vi "setKey.vi"(7 "LegendProperties":T1={"Appearance"={"layout"="", "text-sample order"="", "key order"="", "surroundingBox"=""}, "Alignment"={"Horizontal"="", "Vertical"=""}, "Location"="auto", "\"At\" location"={"XcoordSys"="", "YcoordSys"="", "Xvalue"=0.0, "Yvalue"=0.0}}, 8 "Set?":bool=TRUE, 11 "String in":string) -> (2 "command":string, 3 "String out":string)   [LabVIEW 2013]
uses:
  legendProperties.ctl
  legendAppearance.ctl
  alignment.ctl
  at.ctl
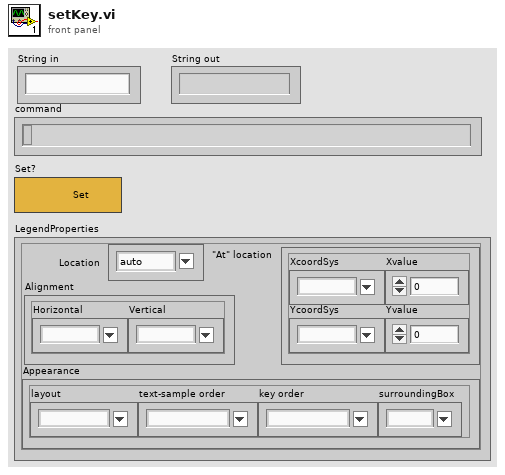
[diagram p1: front panel]
types:
  T1 = typedef "legendProperties.ctl" = cluster{"Appearance":T2, "Alignment":T3, "Location":string, "\"At\" location":T4}
  T2 = typedef "legendAppearance.ctl" = cluster{"layout":string, "text-sample order":string, "key order":string, "surroundingBox":string}
  T3 = typedef "alignment.ctl" = cluster{"Horizontal":string, "Vertical":string}
  T4 = typedef "at.ctl" = cluster{"XcoordSys":string, "YcoordSys":string, "Xvalue":dbl, "Yvalue":dbl}
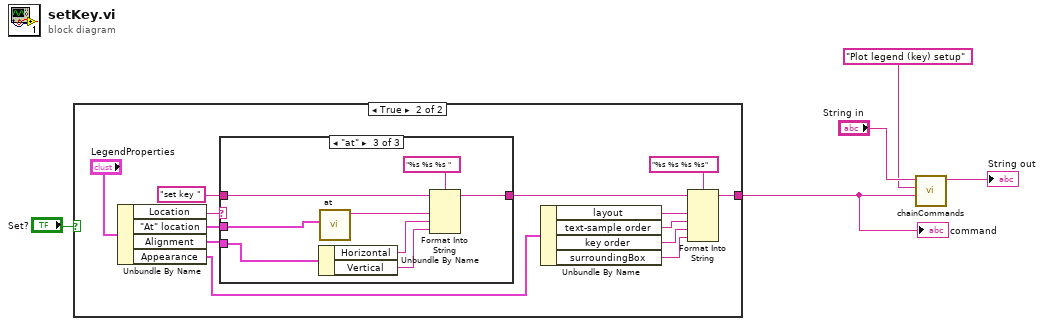
[diagram p0: block diagram]
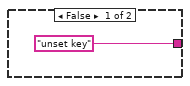
[diagram p2: hidden frame]
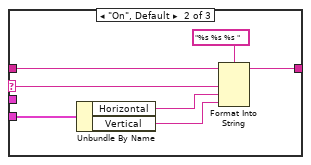
[diagram p4: hidden frame]
diagram:
  n1 = case shown="True" "Set?" {
    tunnel: ["unset key" w17] -> w3
    frame False {
    }
    frame True {
      n2 = Unbundle By Name("LegendProperties") -> ("Location"=w10:string, "\"At\" location"=w9:T4, "Alignment"=w8:T3, "Appearance"=w7:T2)
      n3 = case shown="\"at\"" w10 {
        selector: w10 -> [_ w21 _]
        tunnel: [w20 w27 w35] -> w16
        tunnel: "set key " -> [w20 w26 w34]
        tunnel: w8 -> [_ w22 w29]
        tunnel: w9 -> [_ _ w28]
        frame "auto" {
        }
        frame "On", Default {
          n4 = Unbundle By Name(w22) -> ("Horizontal"=w23:string, "Vertical"=w24:string)
          n5 = Format Into String(format string="%s %s %s ", initial string=w26, w21, w23, w24) -> (resulting string=w27:string)  [unwired: 1 in, 1 out]
        }
        frame "at" {
          n6 = Unbundle By Name(w29) -> ("Horizontal"=w30:string, "Vertical"=w31:string)
          n7 = call "at.vi"("\"At\" location"=w28) -> ("String out"=w32:string)  [unwired: 10 in]
          n8 = Format Into String(format string="%s %s %s ", initial string=w34, w32, w30, w31) -> (resulting string=w35:string)  [unwired: 1 in, 1 out]
        }
      }
      n9 = Unbundle By Name(w7) -> ("layout"=w15:string, "text-sample order"=w14:string, "key order"=w13:string, "surroundingBox"=w12:string)
      n10 = Format Into String(format string="%s %s %s %s", initial string=w16, w15, w14, w13, w12) -> (resulting string=w17:string)  [unwired: 1 in, 1 out]
    }
  }
  "command" <- w3
  n11 = call "chainCommands.vi"("Command"=w3, "Comments"="Plot legend (key) setup", "StringIn"="String in") -> ("StringOut"=→"String out":string)  [unwired: 8 in]
